vi "KeyUp.vi"(1 "Virtual Key":u8(ring)=65) -> ()   [LabVIEW 2009]
uses:
  user32.dll
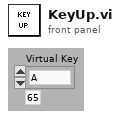
[diagram p1: front panel]
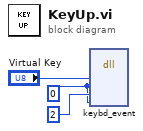
[diagram p0: block diagram]
diagram:
  w2 = u8 0 ("bScan")
  n1 = dll-call lib="user32.dll" fn="keybd_event"("bVk"="Virtual Key", "bScan"=w2, "dwFlags"=u32 2, "dwExtraInfo"=w2) -> ()  [unwired: 8 in, 2 out]
